vi "Threshold Filter.vi"() -> ()   [LabVIEW 2018]
uses:
  <vilib>/Utility/file.llb/Write Delimited Spreadsheet (DBL).vi
panel:
  in  "Save Button":bool
  in  "Stop Button":bool
  in  "Vertical thershhold":dbl(slide)=0.1 scale=0.0..1.0
  in  "Horizontal window":dbl(slide)=50.0 scale=0.0..100.0
  in  "Y col":i32=3
  in  "X col":i32
  out "XY Graph":cluster{"all rows":dbl[], "all rows":dbl[]}[](graph)
  out "Array - Numeric":dbl[][](array[numeric])
  in  "File Path Control":path=path "C:/Data/YD_Q142.013.txt"
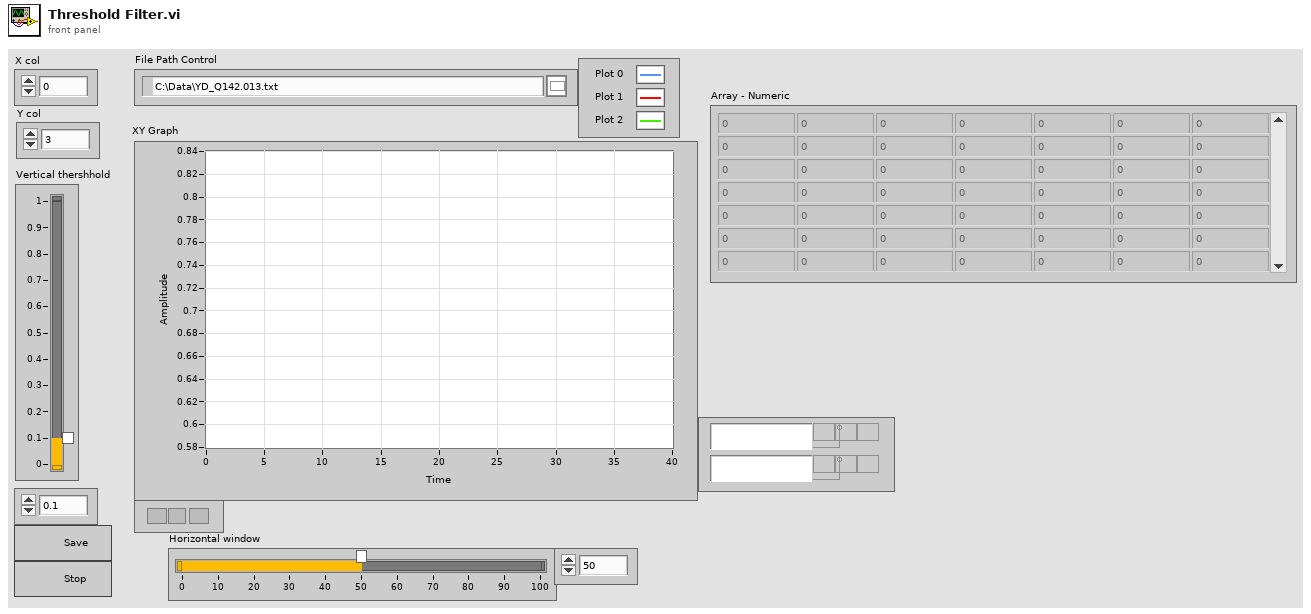
[diagram p1: front panel]
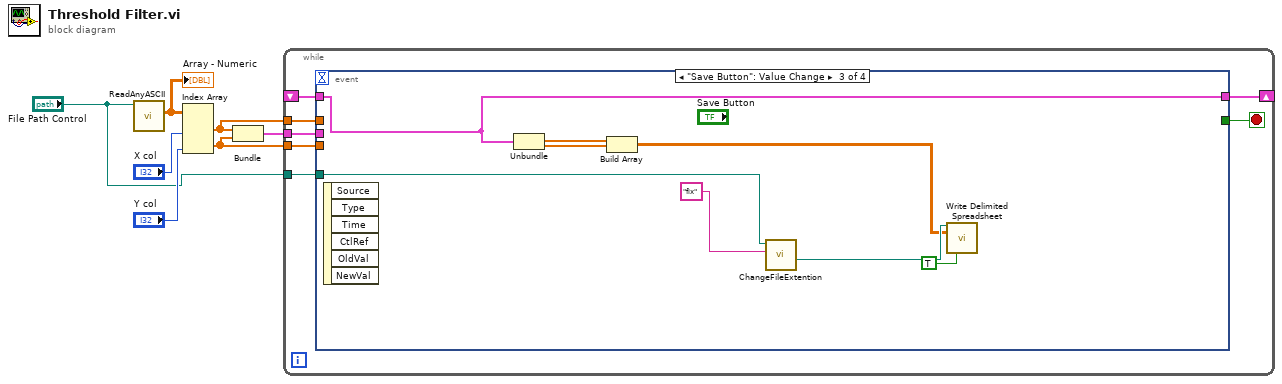
[diagram p0: block diagram]
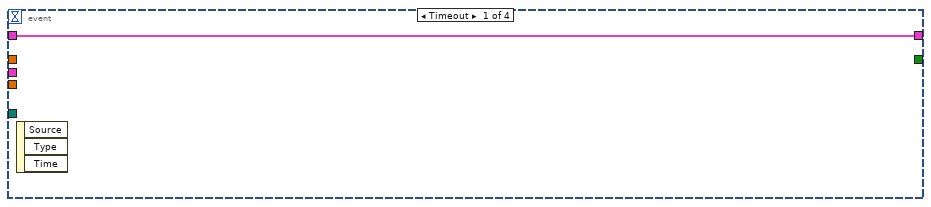
[diagram p2: hidden frame]
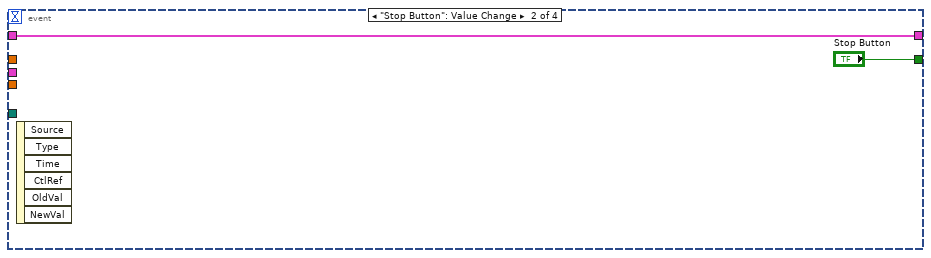
[diagram p3: hidden frame]
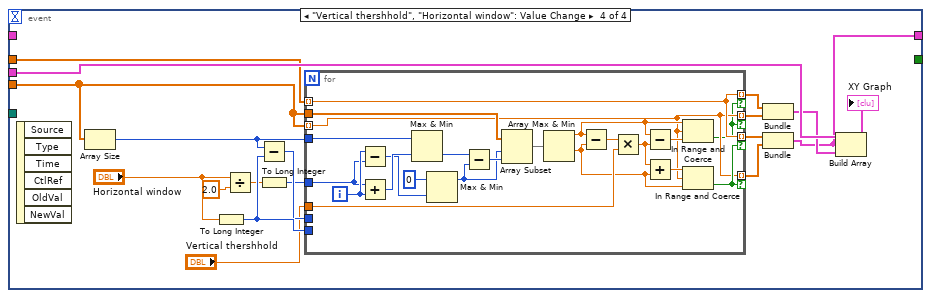
[diagram p4: hidden frame]
diagram:
  n1 = call "ReadAnyASCII.vi"("file path (dialog if empty)"="File Path Control") -> ("all rows"=w7:dbl[][])  [unwired: 8 in, 2 out]
  "Array - Numeric" <- w7
  n2 = Index Array(array=w7, index (col) #1="X col", index (col) #2="Y col") -> (element #1=w2:dbl[], element #2=w3:dbl[])  [unwired: 2 in]
  n3 = Bundle("all rows"=w2, "all rows"=w3) -> (w4:cluster{"all rows":dbl[], "all rows":dbl[]})  [unwired: 1 in]
  n4 = while {
    tunnel: w4 -> [w13]
    tunnel: w3 -> [w12]
    tunnel: w2 -> [w11]
    shift-right: [w10] -> _
    shift-left: _ -> [w9]
    tunnel: "File Path Control" -> [w8]
    stop <- w14 stop-if-true
    n5 = event shown="[2] \"Save Button\": Value Change" {
      selector: _ -> [_ _ _ _]
      dyn-events: _ -> [_ _ _ _]
      timeout: _ -> [_ _ _ _]
      tunnel: [_ "Stop Button" _ _] -> w14
      tunnel: w13 -> [_ _ _ w43]
      tunnel: w12 -> [_ _ _ w34]
      tunnel: w11 -> [_ _ _ w31]
      tunnel: [w15 w16 w18 w26] -> w10
      tunnel: w9 -> [w15 w16 w18 _]
      tunnel: w8 -> [_ _ w25 _]
      event Timeout {
        n6 = event-data() -> ()  [unwired: 1 in, 3 out]
      }
      event "Stop Button": Value Change {
        n7 = event-data() -> ()  [unwired: 1 in, 6 out]
      }
      event "Save Button": Value Change {
        n8 = event-data() -> ()  [unwired: 1 in, 6 out]
        n9 = Unbundle(w18) -> (w22:dbl[], w21:dbl[])
        n10 = Build Array(w22, w21) -> (w20:dbl[][])
        n11 = call "ChangeFileExtention.vi"("New extension"="fix" ("string"), "File Path"=w25) -> ("Path with new extension"=w23:path)  [unwired: 4 in, 5 out]
        n12 = call-poly <vilib>:"Write Delimited Spreadsheet.vi"("file path (dialog if empty)"=w23, "2D data"=w20, "transpose? (no:F)"=TRUE) -> ()  [unwired: 11 in, 2 out]
      }
      event "Vertical thershhold", "Horizontal window": Value Change {
        n13 = event-data() -> ()  [unwired: 1 in, 6 out]
        n14 = Array Size(array=w34) -> (size(s)=w36:i32)
        n15 = To Long Integer(number="Horizontal window") -> (32bit integer=w42:i32)
        n16 = Divide(x="Horizontal window", y=2.0) -> (x/y=w38:dbl)
        n17 = Subtract(x=w36, y=w42) -> (x-y=w41:i32)
        n18 = To Long Integer(number=w38) -> (32bit integer=w37:i32)
        n19 = for {
          tunnel: w34 -> [w65]
          tunnel: w42 -> [_]
          tunnel: w41 -> [_]
          tunnel: w37 -> [w63]
          tunnel: w36 -> [w61]
          tunnel: "Vertical thershhold" -> [w53]
          tunnel: w34 -> [w45] mode=indexing
          tunnel: [w45] -> w32 mode=indexing if=w50
          tunnel: w31 -> [w46] mode=indexing
          tunnel: [w46] -> w30 mode=indexing if=w50
          tunnel: [w46] -> w29 mode=indexing if=w44
          tunnel: [w45] -> w28 mode=indexing if=w44
          i -> [w64]
          n20 = Subtract(x=w64, y=w63) -> (x-y=w59:i32)
          n21 = Add(x=w63, y=w64) -> (x+y=w62:i32)
          n22 = Max & Min(x=w61, y=w62) -> (min(x,y)=w60:i32)  [unwired: 1 out]
          n23 = Max & Min(x=0, y=w59) -> (max(x,y)=w56:i32)  [unwired: 1 out]
          n24 = Subtract(x=w60, y=w56) -> (x-y=w57:i32)
          n25 = Array Subset(array=w65, index=w56, length=w57) -> (w55:dbl[])
          n26 = Array Max & Min(array=w55) -> (max value=w48:dbl, min value=w51:dbl)  [unwired: 2 out]
          n27 = Subtract(x=w48, y=w51) -> (x-y=w54:dbl)
          n28 = Multiply(x=w54, y=w53) -> (x*y=w47:dbl)
          n29 = Subtract(x=w48, y=w47) -> (x-y=w49:dbl)
          n30 = Add(x=w47, y=w51) -> (x+y=w52:dbl)
          n31 = In Range and Coerce(upper limit=w48, x=w45, lower limit=w49) -> (In Range?=w44:bool)  [unwired: 1 out]
          n32 = In Range and Coerce(upper limit=w52, x=w45, lower limit=w51) -> (In Range?=w50:bool)  [unwired: 1 out]
        }
        n33 = Bundle(w29, w28) -> (w27:cluster{dbl[], dbl[]})  [unwired: 1 in]
        n34 = Bundle(w30, w32) -> (w26:cluster{dbl[], dbl[]})  [unwired: 1 in]
        n35 = Build Array(w43, w26, w27) -> (→"XY Graph":cluster{"all rows":dbl[], "all rows":dbl[]}[])
      }
    }
  }
